vi "get all UDP nodes.vi"(5 "allow self?":bool, 7 "allow own eng?":bool, 8 "error in":errorcluster, 11 "editor in":refnum<data-value>) -> (0 "error out":errorcluster, 2 "All UDP refs":refnum<data-value>[](array[refnum]), 3 "editor out":refnum<data-value>)   [LabVIEW 2013, in "TEC editor node.lvclass"]
uses:
  TEC editor node.lvclass
  <vilib>/CEF_TreeControl/Node/NISE_CEF_Node.lvclass/NISE_CEF_Node.ctl
  <vilib>/CEF_TreeControl/Node/ReadParent.vi
  <vilib>/CEF_TreeControl/Node/ReadChildren.vi
  <vilib>/CEF_TreeControl/Node/NISE_CEF_Node.lvclass
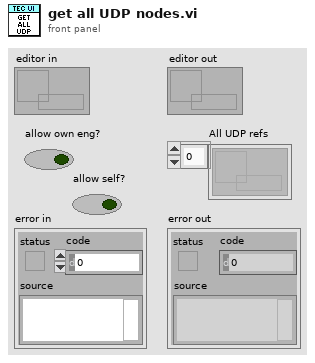
[diagram p1: front panel]
types:
  T1 = typedef "NISE_CEF_Node.lvclass/NodeRef.ctl" = refnum<data-value>
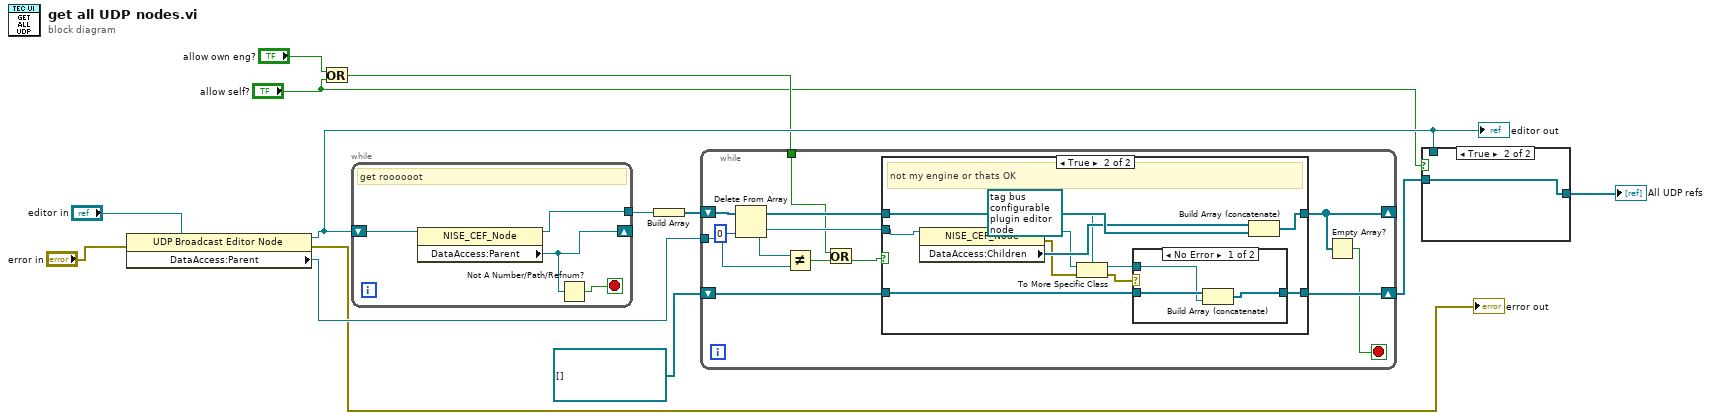
[diagram p0: block diagram]
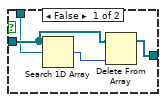
[diagram p2: hidden frame]
diagram:
  n1 = property class="UDP Broadcast Editor Node"(reference="editor in", error in="error in") -> (reference out=w4:refnum<data-value>, error out=→"error out":errorcluster, "DataAccess:Parent"=w9:T1)
  "editor out" <- w4
  n2 = Or(x="allow own eng?", y="allow self?") -> (x .or. y?=w2:bool)
  n3 = while {
    shift-right: [w15] -> _
    shift-left: w4 -> [w17]
    tunnel: [w14] -> w11
    stop <- w16 stop-if-true
    # "get roooooot"
    n4 = property class="NISE_CEF_Node"(reference=w17) -> (reference out=w14:T1, "DataAccess:Parent"=w15:T1)  [unwired: 1 in, 1 out]
    n5 = Not A Number/Path/Refnum?(number/path/refnum=w15) -> (NaN/Path/Refnum?=w16:bool)
  }
  n6 = Build Array(w11) -> (w10:T1[])
  n7 = while {
    shift-right: [w22] -> _
    shift-left: w10 -> [w29]
    tunnel: w9 -> [w27]
    shift-right: [w24] -> w6
    shift-left: refnum<data-value>[] [] ("All UDP refs") -> [w23]
    tunnel: w2 -> [w18]
    stop <- w21 stop-if-true
    n8 = Delete From Array(array=w29, index=0) -> (deleted portion=w20:T1, array with subset deleted=w25:T1[])  [unwired: 1 in]
    n9 = Not Equal?(x=w20, y=w27) -> (x != y?=w26:bool)
    n10 = Or(x=w18, y=w26) -> (x .or. y?=w19:bool)
    n11 = case shown="True" w19 {
      tunnel: w25 -> [w31 w42]
      tunnel: [w31 w41] -> w22
      tunnel: [w30 w32] -> w24
      tunnel: w23 -> [w30 w33]
      tunnel: w20 -> [_ w40]
      frame False {
        # "is my engine"
      }
      frame True {
        # "not my engine or thats OK"
        n12 = property class="NISE_CEF_Node"(reference=w40) -> (reference out=w38:T1, error out=w37:errorcluster, "DataAccess:Children"=w39:T1[])  [unwired: 1 in]
        n13 = To More Specific Class(target class=refnum<data-value> refnum ("UDP refs"), reference=w38, error in=w37) -> (specific class reference=w35:refnum<data-value>, error out=w34:errorcluster)
        n14 = case shown="No Error" w34 {
          tunnel: w35 -> [w44 _]
          tunnel: w33 -> [w45 w46]
          tunnel: [w43 w46] -> w32
          frame No Error {
            n15 = Build Array (concatenate)(w45, w44) -> (w43:refnum<data-value>[])
          }
          frame Error {
          }
        }
        n16 = Build Array (concatenate)(w39, w42) -> (w41:T1[])
      }
    }
    n17 = Empty Array?(array=w22) -> (empty?=w21:bool)
  }
  n18 = case shown="True" "allow self?" {
    tunnel: w6 -> [w50 w51]
    tunnel: [w48 w51] -> w5
    tunnel: w4 -> [w47 _]
    frame False {
      n19 = Search 1D Array(1D array=w50, element=w47) -> (index of element=w49:i32)  [unwired: 1 in]
      n20 = Delete From Array(array=w50, index=w49) -> (array with subset deleted=w48:refnum<data-value>[])  [unwired: 1 in, 1 out]
    }
    frame True {
    }
  }
  "All UDP refs" <- w5
